vi "Service Request Enable.vi"(0 "VISA resource name":refnum<visa-resource-name>, 5 "Service Request Enable":T1, 11 "error in (no error)":errorcluster) -> (4 "VISA resource name out":refnum<visa-resource-name>, 15 "error out":errorcluster)   [LabVIEW 2018, in "XP Power PLS600.lvlib"]
doc: "Controls Service Request enable register which bits from the Status Byte should be used to generate a service request when the bit value = 1.\n\nThe Service Request Enable Register consists of the following 8 bits.\n\nBIT 0: Reserved\nBIT 1: Reserved\nBIT 2: Error in Queue\nBIT 3: QUES = Questionable Status Summary\nBIT 4: MAV = Message Available\nBIT 5: ESB = Event Status Byte Summary\nBIT 6: RQS = Request for Service\nBIT 7: OPER = Operation Event Summary\n\nExample:\n\nIf the user wants to generate SRQ(Service Request) when there is a Message Available and Error in the Queue only, the binary mask 00010100 (0x14) should be used."
uses:
  XP Power PLS600.lvlib
panel:
  # "BIT 0: Reserved\nBIT 1: Reserved\nBIT 2: Error in Queue\nBIT 3: QUES = Questionable Status Summary\nBIT 4: MAV = Message Available\nBIT 5: ESB = Event Status Byte Summary\nBIT 6: RQS = Request for Service\nBIT 7: OPER = Operation Event Summary"
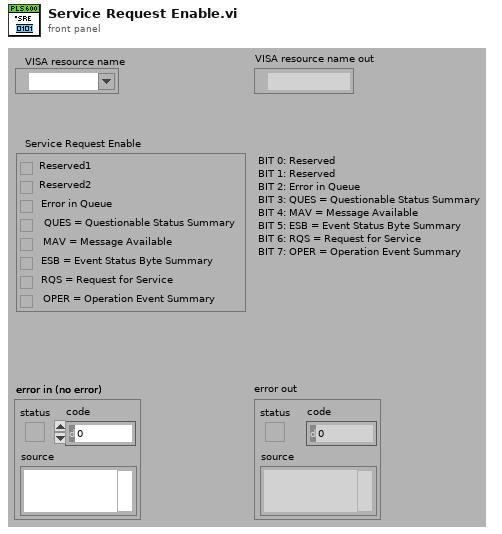
[diagram p1: front panel]
types:
  T1 = cluster{"Reserved1":bool, "Reserved2":bool, "Error in Queue":bool, "QUES = Questionable Status Summary":bool, "MAV = Message Available":bool, "ESB = Event Status Byte Summary":bool, "RQS = Request for Service":bool, "OPER = Operation Event Summary":bool}
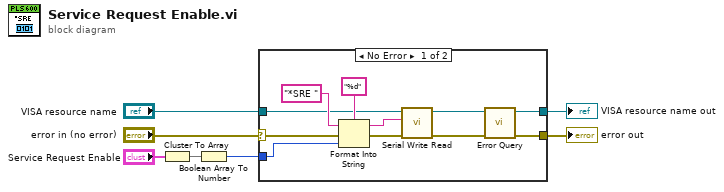
[diagram p0: block diagram]
diagram:
  n1 = Cluster To Array(cluster="Service Request Enable") -> (array=w3:bool[])
  n2 = Boolean Array To Number(Boolean array=w3) -> (number=w1:u32)
  n3 = case shown="No Error" "error in (no error)" {
    selector: "error in (no error)" -> [w16 w19]
    tunnel: w1 -> [w18 _]
    tunnel: "VISA resource name" -> [w12 w20]
    tunnel: [w9 w20] -> w4
    tunnel: [w10 w19] -> w5
    frame No Error {
      n4 = Format Into String(format string="%d", initial string="*SRE " ("Command to Send"), error in=w16, w18) -> (resulting string=w8:string, error out=w11:errorcluster)
      n5 = call "Serial Write Read.vi"("error in (no error)"=w11, "Write Buffer"=w8, "VISA resource name"=w12) -> ("error out"=w14:errorcluster, "VISA resource name out"=w13:refnum<visa-resource-name>)  [unwired: 6 in, 1 out]
      n6 = call "Error Query.vi"("error in (no error)"=w14, "VISA resource name"=w13) -> ("error out"=w10:errorcluster, "VISA resource name out"=w9:refnum<visa-resource-name>)  [unwired: 6 in, 2 out]
    }
    frame Error {
    }
  }
  "error out" <- w5
  "VISA resource name out" <- w4
